vi "HumanExecute.vi"(8 "error in (no error)":errorcluster) -> (0 "error out":errorcluster)   [LabVIEW 2023]
doc: "Execute for Human\n\ninput:\n error in (cluster)\n\noutput:\n error out (cluster)"
uses:
  <vilib>/Rock Robotics/WPI/Joystick/XBox Buttons Indexer.ctl
  <vilib>/Rock Robotics/WPI/Joystick/XBox Axes Indexer.ctl
  <vilib>/Rock Robotics/WPI/ThirdParty/JAS_Junk/TrajLib/MathUtil_ApplyDeadband.vi
  <vilib>/Rock Robotics/WPI/ThirdParty/JAS_Junk/TrajLib/VI/DigSeqLogic_Edge_On.vi
  HumanGlobal.vi
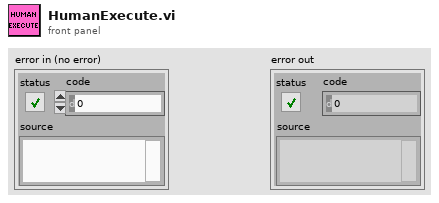
[diagram p1: front panel]
types:
  T1 = typedef "XBox Axes Indexer.ctl" = enum16{"Left X", "Left Y", "Left Trigger", "Right Trigger", "Right X", "Right Y"}
  T2 = typedef "XBox Buttons Indexer.ctl" = enum16{"A", "B", "X", "Y", "Left Bumper", "Right Bumper", "Back", "Start", "Left Joystick", "Right Joystick"}
  T3 = typedef "WPI_JoystickDevRef.ctl" = cluster{"Device":T4}
  T4 = typedef "WPI_JoystickDeviceEnum.ctl" = enum16{"USB 0", "USB 1", "USB 2", "USB 3", "USB 4", "USB 5"}
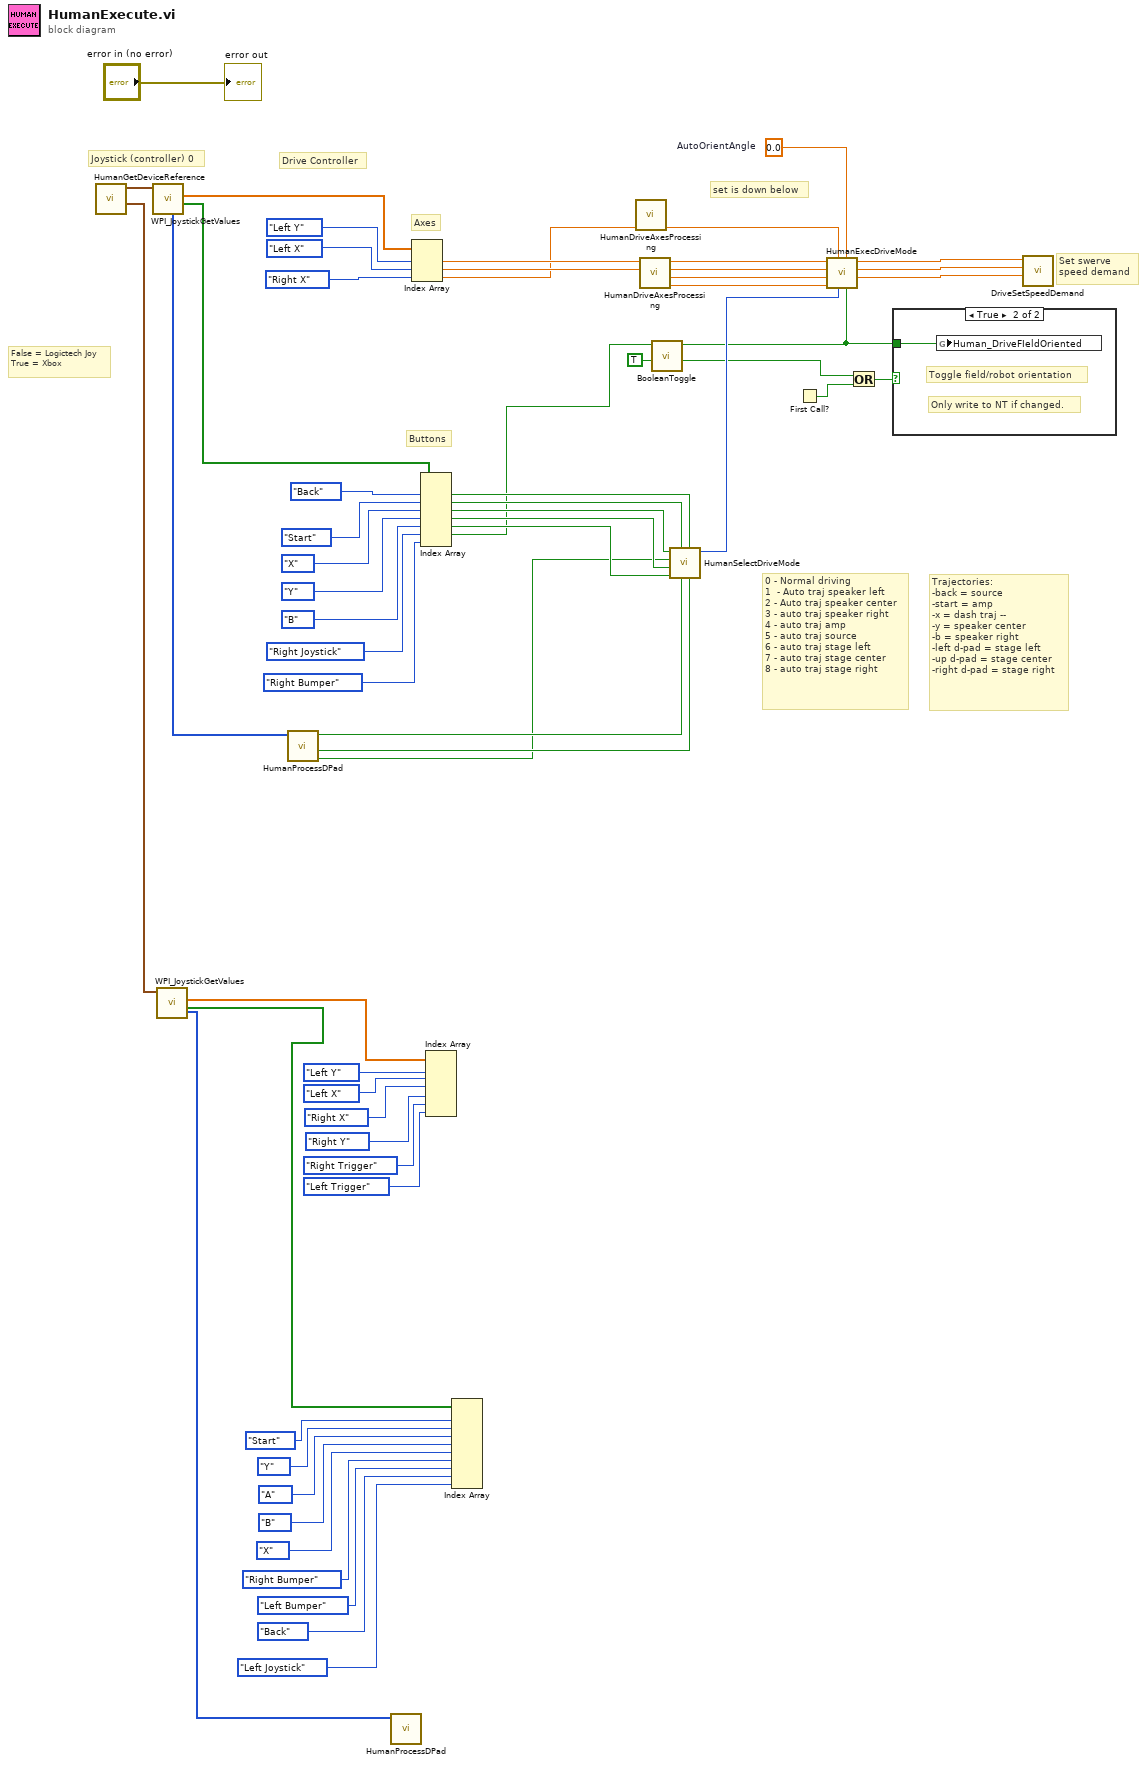
[diagram p0: block diagram]
diagram:
  w1 = 0.0  # AutoOrientAngle
  # "0 - Normal driving\n1  - Auto traj speaker left \n2 - Auto traj speaker center\n3 - auto traj speaker right \n4 - auto traj amp\n5 - auto traj source\n6 - auto traj stage left\n7 - auto traj stage center\n8 - auto traj stage right"
  # "False = Logictech Joy\nTrue = Xbox"
  # "Trajectories:\n-back = source\n-start = amp\n-x = dash traj -- \n-y = speaker center\n-b = speaker right\n-left d-pad = stage left\n-up d-pad = stage center\n-right d-pad = stage right"
  # "Buttons"
  # "Axes"
  # "set is down below"
  # "Set swerve\nspeed demand"
  # "Joystick (controller) 0"
  # "Drive Controller"
  n1 = call "HumanGetDeviceReference.vi"() -> ("Aux Joy"=w47:T3, "Driver Joy"=w51:T3)  [unwired: 9 in, 1 out]
  n2 = call <vilib>:"WPI_JoystickGetValues.vi"("JoystickDevRef"=w51) -> ("Buttons"=w32:bool[], "Axes"=w33:dbl[], "POVs"=w60:i16[])  [unwired: 6 in, 2 out]
  n3 = call <vilib>:"WPI_JoystickGetValues.vi"("JoystickDevRef"=w47) -> ("Buttons"=w37:bool[], "Axes"=w46:dbl[], "POVs"=w26:i16[])  [unwired: 6 in, 2 out]
  n4 = call "HumanProcessDPad.vi"("POV"=w60) -> ("Right"=w18:bool, "Left"=w19:bool, "Up"=w20:bool)  [unwired: 7 in, 1 out]
  n5 = call "HumanProcessDPad.vi"("POV"=w26) -> ()  [unwired: 7 in, 4 out]
  n6 = Index Array(array=w33, index #1=XBox_Axes_Indexer."Left Y" ("XBox Axes"), index #2=XBox_Axes_Indexer."Left X" ("XBox Axes"), index #3=XBox_Axes_Indexer."Right X" ("XBox Axes")) -> (element #1=w59:dbl, element #2=w58:dbl, element #3=w12:dbl)
  n7 = Index Array(array=w32, index #1=XBox_Buttons_Indexer."Back" ("Nothing"), index #2=XBox_Buttons_Indexer."Start" ("Nothing"), index #3=XBox_Buttons_Indexer."X" ("Nothing"), index #4=XBox_Buttons_Indexer."Y" ("Nothing"), index #5=XBox_Buttons_Indexer."B" ("Nothing"), index #6=XBox_Buttons_Indexer."Right Joystick" ("Nothing"), index #7=XBox_Buttons_Indexer."Right Bumper" ("Nothing")) -> (element #1=w25:bool, element #2=w24:bool, element #3=w23:bool, element #4=w22:bool, element #5=w21:bool, element #6=w5:bool)  [unwired: 1 out]
  n8 = Index Array(array=w46, index #1=XBox_Axes_Indexer."Left Y" ("XBox Axes"), index #2=XBox_Axes_Indexer."Left X" ("XBox Axes"), index #3=XBox_Axes_Indexer."Right X" ("XBox Axes"), index #4=XBox_Axes_Indexer."Right Y" ("XBox Axes"), index #5=XBox_Axes_Indexer."Right Trigger" ("XBox Axes"), index #6=XBox_Axes_Indexer."Left Trigger" ("XBox Axes")) -> ()  [unwired: 6 out]
  n9 = Index Array "Index Array"(array=w37, index #1=XBox_Buttons_Indexer."Start" ("Nothing"), index #2=XBox_Buttons_Indexer."Y" ("OpenCloseClaw"), index #3=XBox_Buttons_Indexer."A" ("GrabberIn"), index #4=XBox_Buttons_Indexer."B" ("GrabberOut"), index #5=XBox_Buttons_Indexer."X" ("Nothing"), index #6=XBox_Buttons_Indexer."Right Bumper" ("Nothing"), index #7=XBox_Buttons_Indexer."Left Bumper" ("Nothing"), index #8=XBox_Buttons_Indexer."Back" ("Place Cone"), index #9=XBox_Buttons_Indexer."Left Joystick" ("Place Cone")) -> ()  [unwired: 9 out]
  n10 = call "HumanDriveAxesProcessing.vi"("Right X"=w12) -> ("Right X"=w14:dbl)  [unwired: 7 in, 3 out]
  n11 = call "HumanDriveAxesProcessing.vi"("Left X"=w58, "Left Y"=w59) -> ("Right X"=w11:dbl, "Right Y"=w56:dbl, "Left X"=w57:dbl, "Left Y"=w55:dbl)  [unwired: 6 in]
  n12 = call "BooleanToggle.vi"("InitialState"=TRUE, "Toggle Edge In"=w5) -> ("Changed"=w2:bool, "Output"=w4:bool)  [unwired: 8 in]
  n13 = call "HumanSelectDriveMode.vi"("AutoTrajStageLeft"=w19, "AutoTrajSource"=w25, "AutoTrajStageCenter"=w20, "AutoTrajAmp"=w24, "AutoTrajSpeakerRight"=w21, "AutoTrajSpeakerCenter"=w22, "AutoTrajStageRight"=w18, "AutoTrajSpeakerLeft"=w23) -> ("Drive Mode"=w17:i32)  [unwired: 3 in]
  n14 = First Call?() -> (First Call?: T/F=w6:bool)
  n15 = call "HumanExecDriveMode.vi"("Enable Field Oriented Drive"=w4, "AutoOrientAngle"=w1, "State"=w17, "Rotation"=w14, "Right X"=w11, "Right Y"=w56, "Left X"=w57, "Left Y"=w55) -> ("AMotorDemand"=w54:dbl, "YMotorDemand"=w53:dbl, "XMotorDemand"=w52:dbl)  [unwired: 1 in]
  n16 = Or(x=w2, y=w6) -> (x .or. y?=w7:bool)
  n17 = case shown="True" w7 {
    tunnel: w4 -> [_ w62]
    frame False {
    }
    frame True {
      # "Only write to NT if changed."
      # "Toggle field/robot orientation"
      n18 = global write "HumanGlobal.vi" "Human_DriveFIeldOriented"(w62) -> ()
    }
  }
  n19 = call "DriveSetSpeedDemand.vi"("ASpeedDemand (d/s)"=w54, "YSpeedDemand (ft/s)"=w53, "XSpeedDemand (ft/s)"=w52) -> ()  [unwired: 9 in]
  "error out" <- "error in (no error)"
